vi "Configure Wait Time.vi"(0 "VISA resource name":refnum<visa-resource-name>, 1 "Enable Wait Time (T: Enable)":bool=TRUE, 2 "Auto Set Wait Time (T: Enable)":bool=TRUE, 5 "Channel (0: Channel 1)":i32(ring) items=["Channel 1", "Channel 2"], 7 "Wait Time Gain (1)":dbl=1.0, 9 "Wait Time Offset (0)":dbl, 11 "error in (no error)":errorcluster, 12 "Wait Time Mode (0: Source Wait Time)":i32(ring) items=["Source Wait Time", "Measurement Wait Time"]) -> (4 "VISA resource name out":refnum<visa-resource-name>, 15 "error out":errorcluster)   [LabVIEW 2020, in "Agilent B2900 Series.lvlib"]
doc: "Change settings for source/measurement wait time."
uses:
  Agilent B2900 Series.lvlib
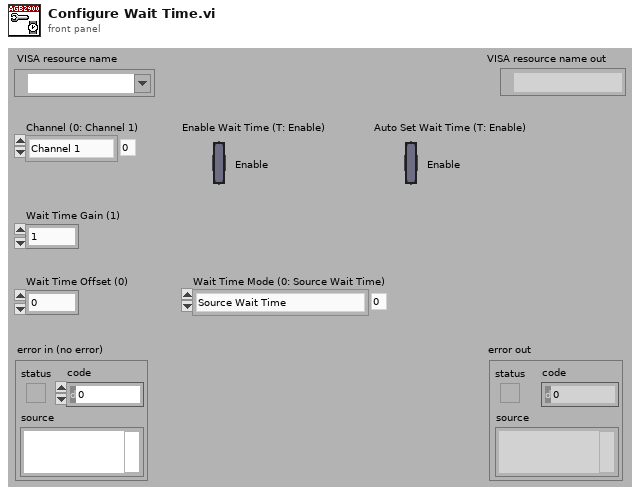
[diagram p1: front panel]
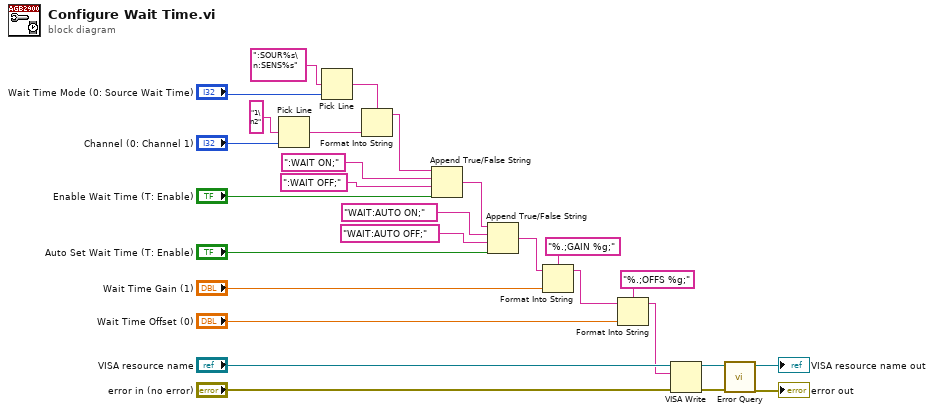
[diagram p0: block diagram]
diagram:
  n1 = Pick Line(multi-line string="1\n2" ("string (\"\")"), line index="Channel (0: Channel 1)") -> (output string=w4:string)  [unwired: 1 in]
  n2 = Pick Line(multi-line string=":SOUR%s\n:SENS%s", line index="Wait Time Mode (0: Source Wait Time)") -> (output string=w5:string)  [unwired: 1 in]
  n3 = Format Into String(format string=w5, w4) -> (resulting string=w3:string)  [unwired: 2 in, 1 out]
  n4 = Append True/False String(1:"Enable Wait Time (T: Enable)", 2:":WAIT OFF;", 3:":WAIT ON;", 4:w3) -> (0:w2:string)
  n5 = Append True/False String(1:"Auto Set Wait Time (T: Enable)", 2:"WAIT:AUTO OFF;", 3:"WAIT:AUTO ON;", 4:w2) -> (0:w24:string)
  n6 = Format Into String(format string="%.;GAIN %g;", initial string=w24, "Wait Time Gain (1)") -> (resulting string=w21:string)  [unwired: 1 in, 1 out]
  n7 = Format Into String(format string="%.;OFFS %g;", initial string=w21, "Wait Time Offset (0)") -> (resulting string=w1:string)  [unwired: 1 in, 1 out]
  n8 = VISA Write(VISA resource name="VISA resource name", write buffer=w1, error in (no error)="error in (no error)") -> (VISA resource name out=w13:refnum<visa-resource-name>, error out=w12:errorcluster)  [unwired: 1 out]
  n9 = call "Error Query.vi"("error in (no error)"=w12, "VISA resource name"=w13) -> ("error out"=→"error out":errorcluster, "VISA resource name out"=→"VISA resource name out":refnum<visa-resource-name>)  [unwired: 6 in, 2 out]
